vi "connectTcpClientA.vi"(8 "error in (no error)":errorcluster) -> (0 "error out":errorcluster, 2 "tel connection ID A out":refnum<k5>, 3 "cmd connection ID A out":refnum<k5>)   [LabVIEW 2018]
doc: "Create the connection ID for TCP client A."
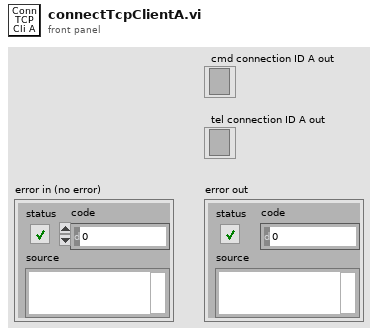
[diagram p1: front panel]
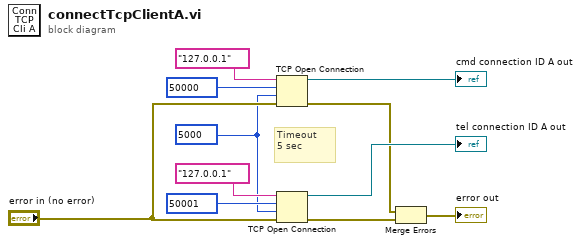
[diagram p0: block diagram]
diagram:
  w4 = 5000 ("timeout ms (60000)")
  # "Timeout\n5 sec"
  n1 = TCP Open Connection(address="127.0.0.1", remote port or service name=u16 50000, timeout ms (60000)=w4, error in (no error)="error in (no error)") -> (connection ID=→"cmd connection ID A out":refnum<k5>, error out=w3:errorcluster)  [unwired: 1 in]
  n2 = TCP Open Connection(address="127.0.0.1", remote port or service name=u16 50001, timeout ms (60000)=w4, error in (no error)="error in (no error)") -> (connection ID=→"tel connection ID A out":refnum<k5>, error out=w2:errorcluster)  [unwired: 1 in]
  n3 = Merge Errors(w3, w2) -> (→"error out":errorcluster)
